vi "write positions to cvt or reload pico.vi"(8 "error in (no error)":errorcluster, 10 "Array":dbl[](array[numeric]), 11 "Picomotor8742dotNet in":refnum<class "Picomotor8742dotNet.lvclass">) -> (0 "error out":errorcluster, 2 "new command":string, 3 "Picomotor8742dotNet out":refnum<class "Picomotor8742dotNet.lvclass">)   [LabVIEW 2020, in "Picomotor8742dotNet.lvclass"]
uses:
  Picomotor8742dotNet.lvclass
  Picomotor8742dotNet.lvclass/Picomotor8742dotNet.ctl
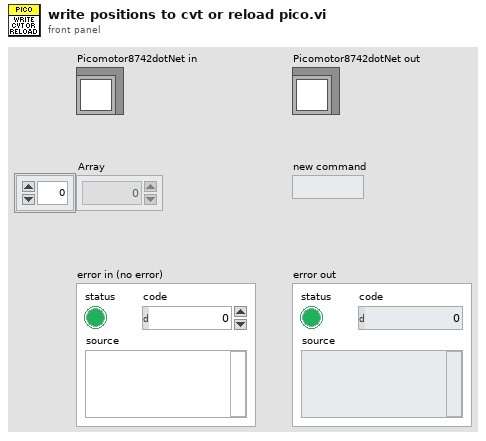
[diagram p1: front panel]
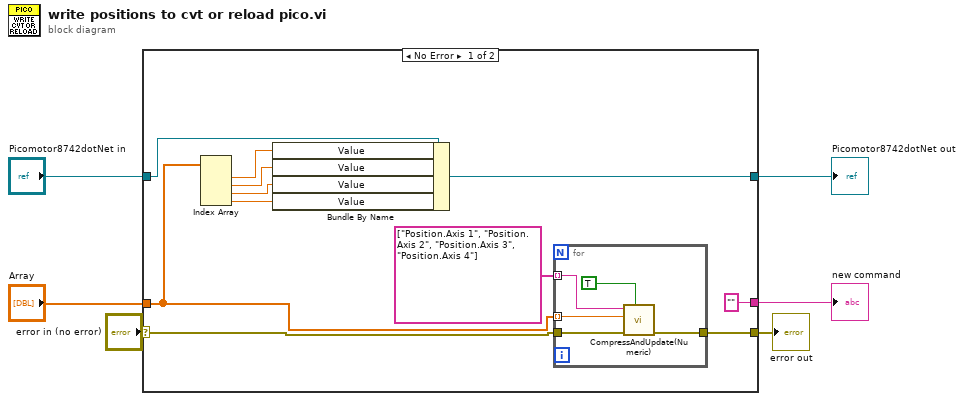
[diagram p0: block diagram]
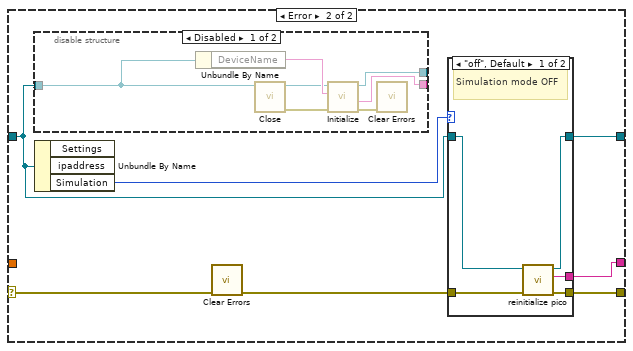
[diagram p2: hidden frame]
diagram:
  n1 = case shown="No Error" "error in (no error)" {
    selector: "error in (no error)" -> [w15 w28]
    tunnel: "Array" -> [w10 _]
    tunnel: [w16 w29] -> w2
    tunnel: "Picomotor8742dotNet in" -> [w8 w24]
    tunnel: [w9 w26] -> w4
    tunnel: ["" ("new command") w25] -> w5
    frame No Error {
      n2 = Index Array(array=w10) -> (element #1=w11:dbl, element #2=w12:dbl, element #3=w13:dbl, element #4=w14:dbl)  [unwired: 4 in]
      n3 = Bundle By Name(cluster=w8, "Value"=w11, "Value"=w12, "Value"=w13, "Value"=w14) -> (w9:refnum<class "Picomotor8742dotNet.lvclass">)
      n4 = for {
        tunnel: w10 -> [w20] mode=indexing
        tunnel: string[] ["Position.Axis 1", "Position.Axis 2", "Position.Axis 3", "Position.Axis 4"] -> [w21] mode=indexing
        tunnel: w15 -> [w19]
        tunnel: [w18] -> w16
        n5 = call "CompressAndUpdate(Numeric).vi"("force CVT update (false)"=TRUE ("force CVT update"), "error in"=w19, "Numeric"=w20, "command or variable name"=w21) -> ("error out"=w18:errorcluster)  [unwired: 7 in]
      }
    }
    frame Error {
      n6 = disable-structure shown="Disabled" {
        disable-tunnel: [w32 w37] -> _
        disable-tunnel: [w31 _] -> _
        disable-tunnel: w24 -> [w30 w37]
        frame Disabled {
          n7 = Unbundle By Name(w30) -> ("DeviceName"=w34:string)
          n8 = call-dynamic "Close.vi"("FakePressureController in"=w30) -> ("error out"=w35:errorcluster, "FakePressureController out"=w33:refnum<class "Picomotor8742dotNet.lvclass">)  [unwired: 7 in, 2 out]
          n9 = call-dynamic "Initialize.vi"("error in (no error)"=w35, "DeviceName"=w34, "Object in"=w33) -> ("error out"=w36:errorcluster, "new command(s)"=w31:string, "Object out"=w32:refnum<class "Picomotor8742dotNet.lvclass">)  [unwired: 5 in, 1 out]
          n10 = call "Clear Errors.vi"("error in (no error)"=w36) -> ()  [unwired: 5 in, 2 out]
        }
        frame Enabled {
        }
      }
      n11 = Unbundle By Name(w24) -> ("Simulation"=w23:enum16{"off", "on"})  [unwired: 2 out]
      n12 = call "Clear Errors.vi"("error in (no error)"=w28) -> ("error out"=w27:errorcluster)  [unwired: 5 in, 1 out]
      n13 = case shown="\"off\", Default" w23 {
        tunnel: w24 -> [w38 w44]
        tunnel: [w42 w44] -> w26
        tunnel: w27 -> [w40 w43]
        tunnel: [w41 w43] -> w29
        tunnel: [w39 _] -> w25
        frame "off", Default {
          # "Simulation mode OFF"
          n14 = call "reinitialize pico.vi"("error in (no error)"=w40, "Picomotor8742dotNet in"=w38) -> ("error out"=w41:errorcluster, "new command"=w39:string, "Picomotor8742dotNet out"=w42:refnum<class "Picomotor8742dotNet.lvclass">)  [unwired: 7 in]
        }
        frame "on" {
          # "Simulation mode ON"
        }
      }
    }
  }
  "new command" <- w5
  "Picomotor8742dotNet out" <- w4
  "error out" <- w2
